vi "Dequeue.vi"(8 "error in (no error)":errorcluster, 9 "Timeout ms (-1)":i32, 11 "MessageQ in":refnum<class "MessageQ.lvclass">) -> (0 "error out":errorcluster, 1 "Data":variant, 2 "ID":string, 3 "MessageQ out":refnum<class "MessageQ.lvclass">)   [LabVIEW 2020, in "Volatus.lvlib" / "MessageQ.lvclass"]
uses:
  MessageQ.lvclass
  MessageQ.lvclass/MessageQ.ctl
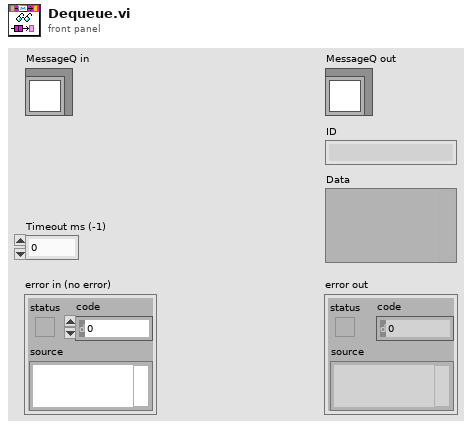
[diagram p1: front panel]
types:
  T1 = typedef "Volatus.lvlib/MessageQ.lvclass/Message.ctl" = cluster{"ID":string, "Data":variant}
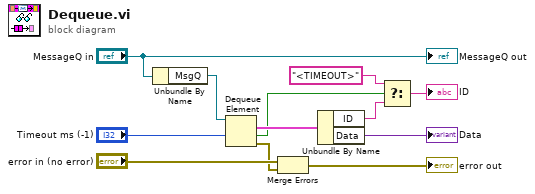
[diagram p0: block diagram]
diagram:
  n1 = Unbundle By Name("MessageQ in") -> ("MsgQ"=w10:refnum<queue>)
  n2 = Dequeue Element(queue=w10, timeout in ms (-1)="Timeout ms (-1)") -> (element=w6:T1, timed out?=w1:bool, error out=w7:errorcluster)  [unwired: 1 in, 1 out]
  n3 = Merge Errors("error in (no error)", w7) -> (→"error out":errorcluster)
  n4 = Unbundle By Name(w6) -> ("ID"=w4:string, "Data"=→"Data":variant)
  n5 = Select(t="<TIMEOUT>", s=w1, f=w4) -> (s? t:f=→"ID":string)
  "MessageQ out" <- "MessageQ in"
